vi "前面板.vi"() -> ()   [LabVIEW 2020]
uses:
  <vilib>/Instr/_visa.llb/VISA Configure Serial Port (Instr).vi
panel:
  in  "下限":dbl
  in  "上限":dbl
  out "错误输出":errorcluster
  in  "确定按钮":bool
  out "运行":bool
  out "警报":bool
  out "当前温度":dbl
  in  "结束":bool
  in  "停止":bool
  out "卡尔曼滤波":dbl(graph)
  out "温度计":dbl(slide) scale=20.0..40.0
  out "原数值波形":dbl(graph)
  in  "串口选择":refnum<visa-resource-name>
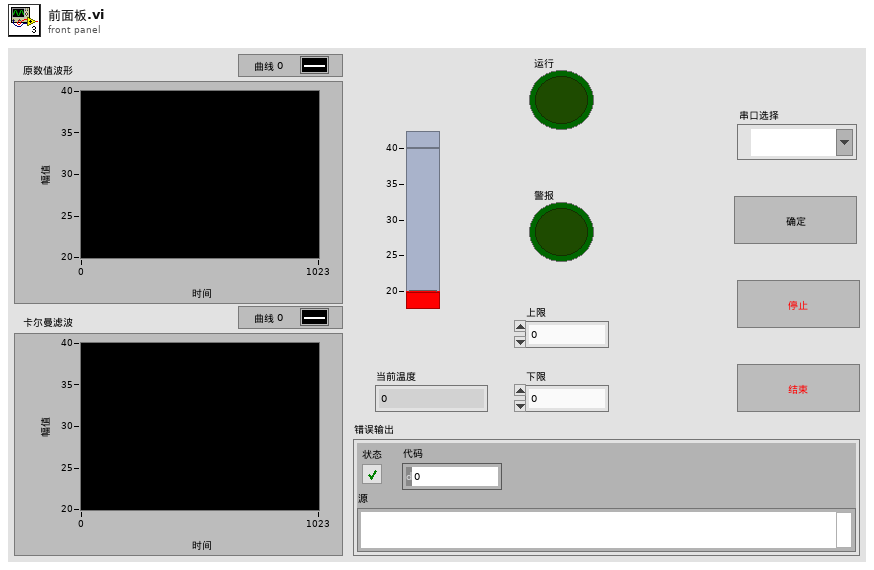
[diagram p1: front panel]
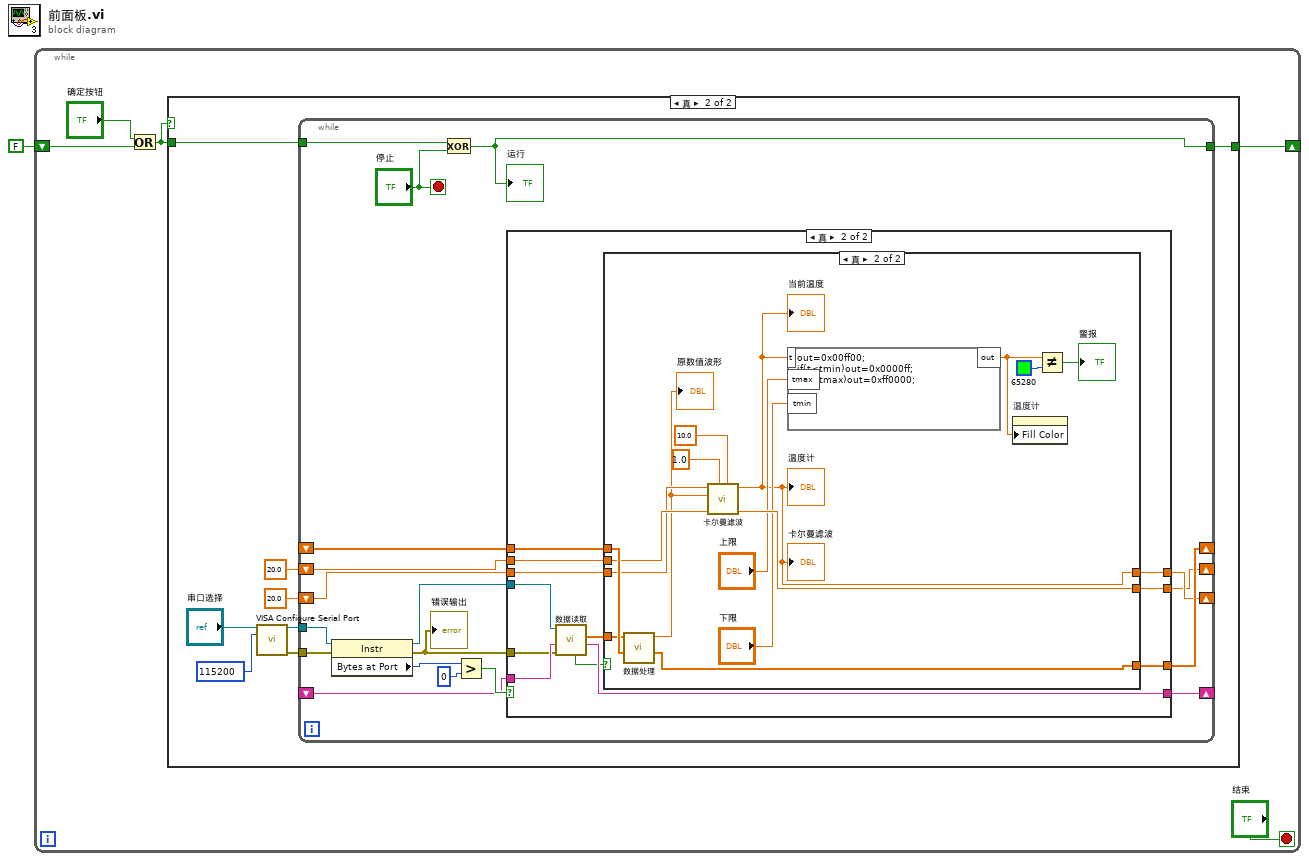
[diagram p0: block diagram]
diagram:
  n1 = while {
    shift-right: [w4] -> _
    shift-left: FALSE -> [w2]
    stop <- "结束" stop-if-true
    n2 = Or(x="确定按钮", y=w2) -> (x .or. y?=w3:bool)
    n3 = case shown="真" w3 {
      tunnel: [w7 w15] -> w4
      tunnel: w3 -> [w7 w14]
      frame False {
      }
      frame True {
        n4 = call-poly "VISA Configure Serial Port"("VISA resource name"="串口选择", "baud rate (9600)"=u32 115200) -> ("VISA resource name out"=w11:refnum<visa-resource-name>, "error out"=w10:errorcluster)  [unwired: 12 in]
        n5 = while {
          tunnel: [w16] -> w15
          tunnel: w14 -> [w28]
          tunnel: w11 -> [w27]
          tunnel: w10 -> [w26]
          shift-right: [w24] -> _
          shift-left: _ -> [w23]
          shift-right: [w22] -> _
          shift-left: 20.0 ("本轮输出") -> [w21]
          shift-right: [w20] -> _
          shift-left: _ -> [w19]
          shift-right: [w17] -> _
          shift-left: 20.0 ("本轮估算协方差") -> [w18]
          stop <- "停止" stop-if-true
          n6 = property class="Instr"(reference=w27, error in=w26) -> (reference out=w33:refnum<visa-resource-name>, error out=w25:errorcluster, "Bytes at Port"=w32:u32)
          "错误输出" <- w25
          n7 = Exclusive Or(1:"停止", 2:w28) -> (0:w16:bool)
          "运行" <- w16
          n8 = Greater?(x=w32, y=u32 0) -> (0:w30:bool)
          n9 = case shown="真" w30 {
            tunnel: w19 -> [w37 w49]
            tunnel: [w37 w48] -> w20
            tunnel: w23 -> [w36 w47]
            tunnel: [w36 w46] -> w24
            tunnel: w25 -> [_ w44]
            tunnel: w33 -> [_ w43]
            tunnel: [w35 w41] -> w22
            tunnel: [w34 w40] -> w17
            tunnel: w18 -> [w34 w39]
            tunnel: w21 -> [w35 w38]
            frame False {
            }
            frame True {
              n10 = call "数据读取.vi"("error out"=w44, "输入字符串"=w49, "VISA resource name out"=w43) -> ("输出字符串"=w48:string, "数组 3"=w45:sgl[], "布尔"=w42:bool)  [unwired: 4 in, 2 out]
              n11 = case shown="真" w42 {
                tunnel: w47 -> [w52 w67]
                tunnel: [w52 w66] -> w46
                tunnel: w45 -> [_ w65]
                tunnel: [w51 w56] -> w41
                tunnel: [w50 w62] -> w40
                tunnel: w39 -> [w50 w61]
                tunnel: w38 -> [w51 w60]
                frame False {
                }
                frame True {
                  n12 = call "数据处理.vi"("输入数组"=w67, "读取数据"=w65) -> ("输出数组"=w66:dbl[], "当前温度"=w59:dbl)  [unwired: 7 in, 1 out]
                  "原数值波形" <- w59
                  n13 = call "卡尔曼滤波.vi"("R"=10.0, "Q"=1.0, "上一轮估算协方差"=w61, "输入"=w59, "上一轮输出"=w60) -> ("本轮估算协方差"=w62:dbl, "本轮输出"=w56:dbl)  [unwired: 5 in]
                  "温度计" <- w56
                  "卡尔曼滤波" <- w56
                  "当前温度" <- w56
                  n14 = formula code="out=0x00ff00;\nif(t<tmin)out=0x0000ff;\nif(t>tmax)out=0xff0000;"("t"=w56, "tmax"="上限", "tmin"="下限") -> ("out"=w53:dbl)
                  n15 = property on="温度计" class="Slide (严格)"("Fill Color"=w53) -> ()  [unwired: 2 in, 2 out]
                  n16 = Not Equal?(x=w53, y=u32 65280) -> (x != y?=→"警报":bool)
                }
              }
            }
          }
        }
      }
    }
  }
